vi "TORC-TapeMeasureAutonomousPID.vi"(10 "Target":dbl) -> ()   [LabVIEW 2014]
doc: "One of the VIs created by TORC 2137 to control the tape measure. Place this within your code's Autonomous Independed.vi.\n\nNote that THIS VI CONTAINS A LOOP.\n\nThis VI will, based on the current and desired position of the tape measure, place a motor speed in a global variable, where it will then be received and used in Periodic Tasks. This VI will run until it reaches the desired target position, at which point the VI will stop and other code will continue.\n\nThere is only one required input; this is the target value for the tape measure. This value is in inches, since the encoder has been calibrated to provide units in inches."
uses:
  TORC-TapeMeasureGlobal.vi
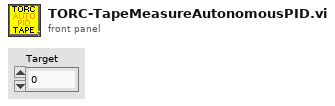
[diagram p1: front panel]
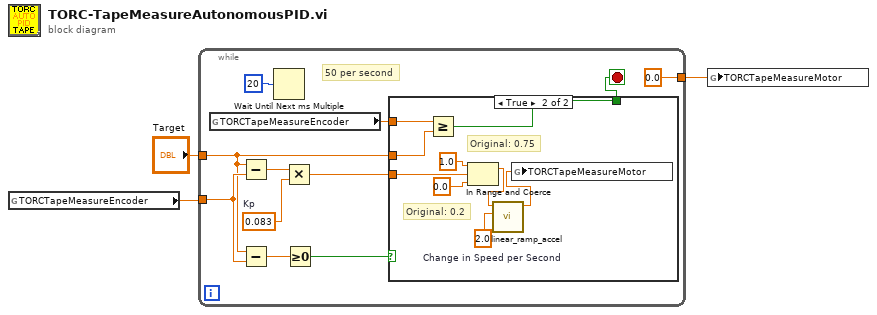
[diagram p0: block diagram]
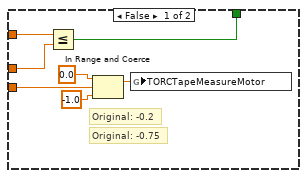
[diagram p2: hidden frame]
diagram:
  n1 = global read "TORC-TapeMeasureGlobal.vi" "TORCTapeMeasureEncoder"() -> (w2:dbl)
  n2 = while {
    tunnel: [0.0 ("LeftMotorValue")] -> w1
    tunnel: w2 -> [w9]
    tunnel: "Target" -> [w5]
    stop <- w12 stop-if-true
    w8 = 0.083  # Kp
    # "50 per second"
    n3 = global read "TORC-TapeMeasureGlobal.vi" "TORCTapeMeasureEncoder"() -> (w4:dbl)
    n4 = Subtract(x=w5, y=w9) -> (x-y=w7:dbl)
    n5 = Subtract(x=w5, y=w9) -> (x-y=w10:dbl)
    n6 = Wait Until Next ms Multiple(millisecond multiple=u32 20) -> ()  [unwired: 1 out]
    n7 = Multiply(x=w7, y=w8) -> (x*y=w6:dbl)
    n8 = Greater Or Equal To 0?(x=w10) -> (x >= 0?=w13:bool)
    n9 = case shown="True" w13 {
      tunnel: w4 -> [w20 w29]
      tunnel: [w21 w30] -> w12
      tunnel: w5 -> [w19 w28]
      tunnel: w6 -> [w18 w27]
      frame False {
        # "Original: -0.2"
        # "Original: -0.75"
        n10 = Less Or Equal?(x=w20, y=w19) -> (x <= y?=w21:bool)
        n11 = In Range and Coerce(upper limit=0.0, x=w18, lower limit=-1.0) -> (coerced(x)=w15:dbl)  [unwired: 1 out]
        n12 = global write "TORC-TapeMeasureGlobal.vi" "TORCTapeMeasureMotor"(w15) -> ()
      }
      frame True {
        w24 = 2.0  # Change in Speed per Second
        # "Original: 0.2"
        # "Original: 0.75"
        n13 = Greater Or Equal?(x=w29, y=w28) -> (x >= y?=w30:bool)
        n14 = In Range and Coerce(upper limit=1.0, x=w27, lower limit=0.0) -> (coerced(x)=w23:dbl)  [unwired: 1 out]
        n15 = call "linear_ramp_accel.vi"("filter const (dx/dt)"=w24, "input"=w23) -> ("output"=w22:dbl)  [unwired: 9 in]
        n16 = global write "TORC-TapeMeasureGlobal.vi" "TORCTapeMeasureMotor"(w22) -> ()
      }
    }
  }
  n17 = global write "TORC-TapeMeasureGlobal.vi" "TORCTapeMeasureMotor"(w1) -> ()
